vi "initializeFont.vi"(8 "error in (no error)":errorcluster, 11 "Font in":refnum<class "Font.lvclass">) -> (0 "error out":errorcluster, 3 "Font out":refnum<class "Font.lvclass">)   [LabVIEW 2020, in "Fonts.lvlib" / "Font.lvclass"]
uses:
  Font.lvclass
  Font.lvclass/Font.ctl
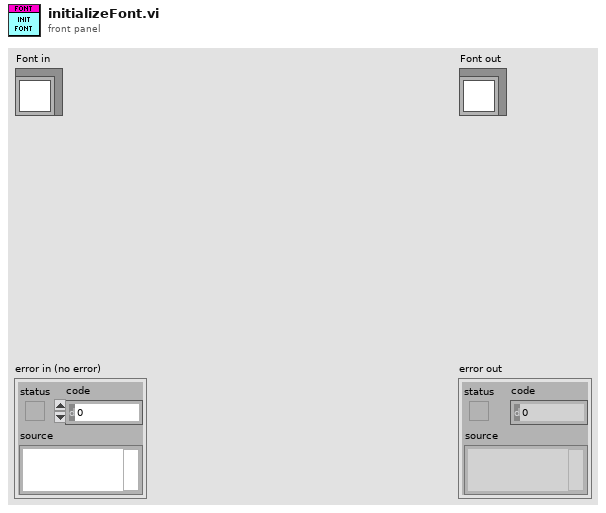
[diagram p1: front panel]
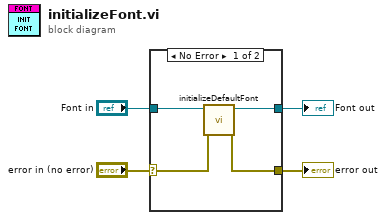
[diagram p0: block diagram]
diagram:
  n1 = case shown="No Error" "error in (no error)" {
    selector: "error in (no error)" -> [w8 w10]
    tunnel: [w6 w10] -> w3
    tunnel: [w5 w9] -> w1
    tunnel: "Font in" -> [w7 w9]
    frame No Error {
      n2 = call-dynamic "initializeDefaultFont.vi"("error in (no error)"=w8, "Font in"=w7) -> ("error out"=w6:errorcluster, "Font out"=w5:refnum<class "Font.lvclass">)  [unwired: 8 in]
    }
    frame Error {
    }
  }
  "error out" <- w3
  "Font out" <- w1
